vi "update.path.vi"() -> (2 "path":string)   [LabVIEW 2020, in "event.lvclass"]
uses:
  event.lvclass
  event.lvclass/event.ctl
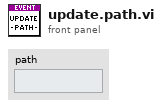
[diagram p1: front panel]
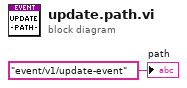
[diagram p0: block diagram]
diagram:
  "path" <- "event/v1/update-event" ("path")
